vi "5.vi"() -> ()   [LabVIEW 2020]
uses:
  #typedef_LogsAction.ctl
  #typedef_Log.ctl
panel:
  in  "stop":bool
  out "List of logs":string
  in  "Limit of logs":i32
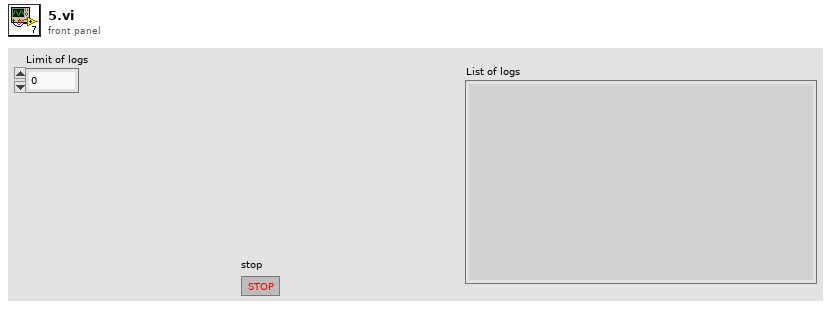
[diagram p1: front panel]
types:
  T1 = typedef "#typedef_LogsAction.ctl" = enum16{"ClearList", "AddRecord", "GetList"}
  T2 = typedef "#typedef_Log.ctl" = cluster{"Info":string, "Time and data of log's registration":timestamp}
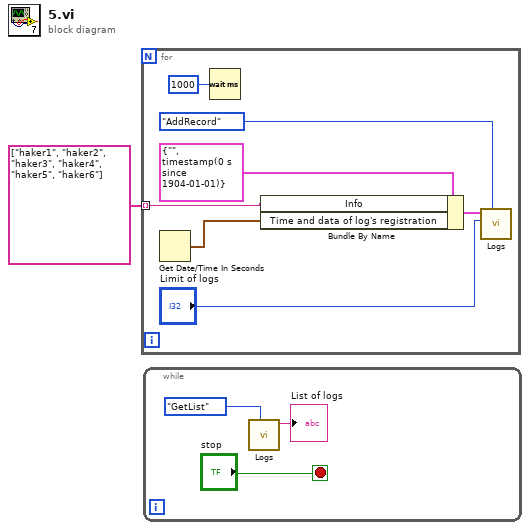
[diagram p0: block diagram]
diagram:
  n1 = for {
    tunnel: string[] ["haker1", "haker2", "haker3", "haker4", "haker5", "haker6"] -> [w5] mode=indexing
    n2 = Get Date/Time In Seconds() -> (seconds since 1Jan1904=w6:timestamp)
    n3 = Wait (ms)(milliseconds to wait=u32 1000) -> ()  [unwired: 1 out]
    n4 = Bundle By Name(cluster=T2 {"Info"="", "Time and data of log's registration"=timestamp(0 s since 1904-01-01)} ("Logs"), "Info"=w5, "Time and data of log's registration"=w6) -> (w8:T2)
    n5 = call "Logs.vi"("Action (GetList)"=#typedef_LogsAction."AddRecord" ("Action"), "Limit of logs"="Limit of logs", "Logs"=w8) -> ()  [unwired: 7 in, 2 out]
  }
  n6 = while {
    stop <- "stop" stop-if-true
    n7 = call "Logs.vi"("Action (GetList)"=#typedef_LogsAction."GetList" ("Action")) -> ("List of logs"=→"List of logs":string)  [unwired: 9 in, 1 out]
  }
